vi "Status Logging.vi"(0 "VISA resource name":refnum<visa-resource-name>, 11 "error in (no error)":errorcluster) -> (4 "VISA resource name out":refnum<visa-resource-name>, 6 "Log Number":dbl min=0.0 max=1500.0 step=1.0, 8 "Logging Status":bool, 15 "error out":errorcluster)   [LabVIEW 2012, in "Lake Shore Cryotronics 218.lvlib"]
doc: "This VI determines if the 218 is actively logging data and what the number is of the last data log record stored."
uses:
  <instrlib>/Lake Shore Cryotronics 218/Lake Shore Cryotronics 218.lvlib
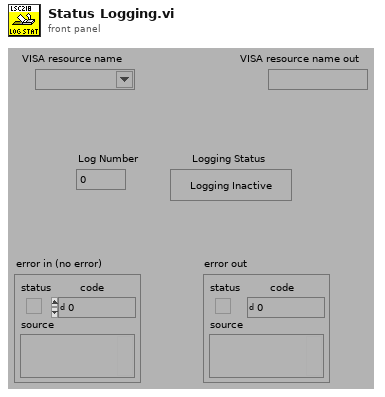
[diagram p1: front panel]
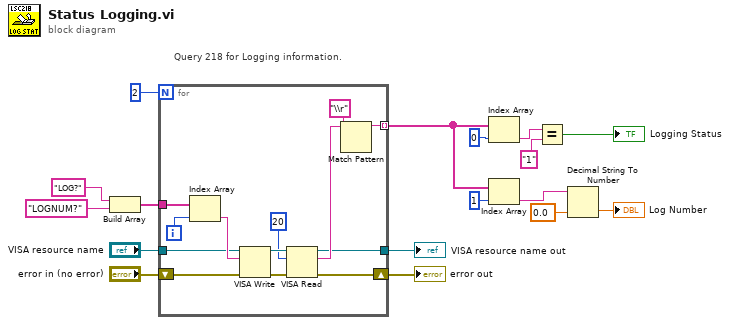
[diagram p0: block diagram]
diagram:
  # "Query 218 for Logging information."
  n1 = Build Array("LOG?", "LOGNUM?") -> (w16:string[])
  n2 = for {
    N: 2 -> [_]
    tunnel: [w26] -> w13 mode=indexing
    shift-right: [w23] -> w2
    shift-left: "error in (no error)" -> [w24]
    tunnel: [w22] -> w5
    tunnel: w16 -> [w20]
    tunnel: "VISA resource name" -> [w19]
    i -> [w25]
    n3 = Index Array(array=w20, index=w25) -> (element=w21:string)
    n4 = VISA Write(VISA resource name=w19, write buffer=w21, error in (no error)=w24) -> (VISA resource name out=w30:refnum<visa-resource-name>, error out=w29:errorcluster)  [unwired: 1 out]
    n5 = VISA Read(VISA resource name=w30, byte count=20, error in (no error)=w29) -> (VISA resource name out=w22:refnum<visa-resource-name>, read buffer=w27:string, error out=w23:errorcluster)  [unwired: 1 out]
    n6 = Match Pattern(string=w27, regular expression="\\r") -> (before substring=w26:string)  [unwired: 1 in, 3 out]
  }
  "VISA resource name out" <- w5
  "error out" <- w2
  n7 = Index Array(array=w13, index=0) -> (element=w12:string)
  n8 = Index Array(array=w13, index=1) -> (element=w9:string)
  n9 = Equal?(x=w12, y="1") -> (x = y?=→"Logging Status":bool)
  n10 = Decimal String To Number(string=w9, default (0L)=0.0) -> (number=→"Log Number":dbl)  [unwired: 1 in, 1 out]
